vi "GetDeviceModel.vi"(8 "error in (no error)":errorcluster) -> (0 "error out":errorcluster, 1 "found":bool, 3 "device model":T1)   [LabVIEW 2017, in "GlobalConfiguration.lvlib"]
doc: "Returns the entire device model, including device properties, channel properties, and tags."
uses:
  <vilib>/addons/InsightCM/Utilities/GlobalConfiguration/GlobalConfiguration.lvlib
  <vilib>/addons/InsightCM/MessageBus/Base/controls/R2_DeviceModel.ctl
  <vilib>/addons/InsightCM/MessageBus/Base/controls/R2_Device.ctl
  <vilib>/addons/InsightCM/MessageBus/Base/controls/KeyValuePair.ctl
  <vilib>/addons/InsightCM/MessageBus/Base/controls/DeviceState.ctl
  <vilib>/addons/InsightCM/MessageBus/Base/controls/R2_DataGroup.ctl
  <vilib>/addons/InsightCM/MessageBus/Base/controls/OperatingState.ctl
  <vilib>/addons/InsightCM/MessageBus/Base/controls/Trigger.ctl
  <vilib>/addons/InsightCM/MessageBus/Base/controls/Condition.ctl
  <vilib>/addons/InsightCM/MessageBus/Base/controls/BurstModeTrigger.ctl
  <vilib>/addons/InsightCM/MessageBus/Base/controls/DeviceSensorGroup.ctl
  <vilib>/addons/InsightCM/MessageBus/Base/controls/Endpoint.ctl
  <vilib>/addons/InsightCM/MessageBus/Base/controls/WirelessChannel.ctl
  <vilib>/addons/InsightCM/MessageBus/Base/controls/R2_Channel.ctl
  <vilib>/addons/InsightCM/MessageBus/Base/controls/Metric.ctl
  <vilib>/addons/InsightCM/MessageBus/Base/controls/Tag.ctl
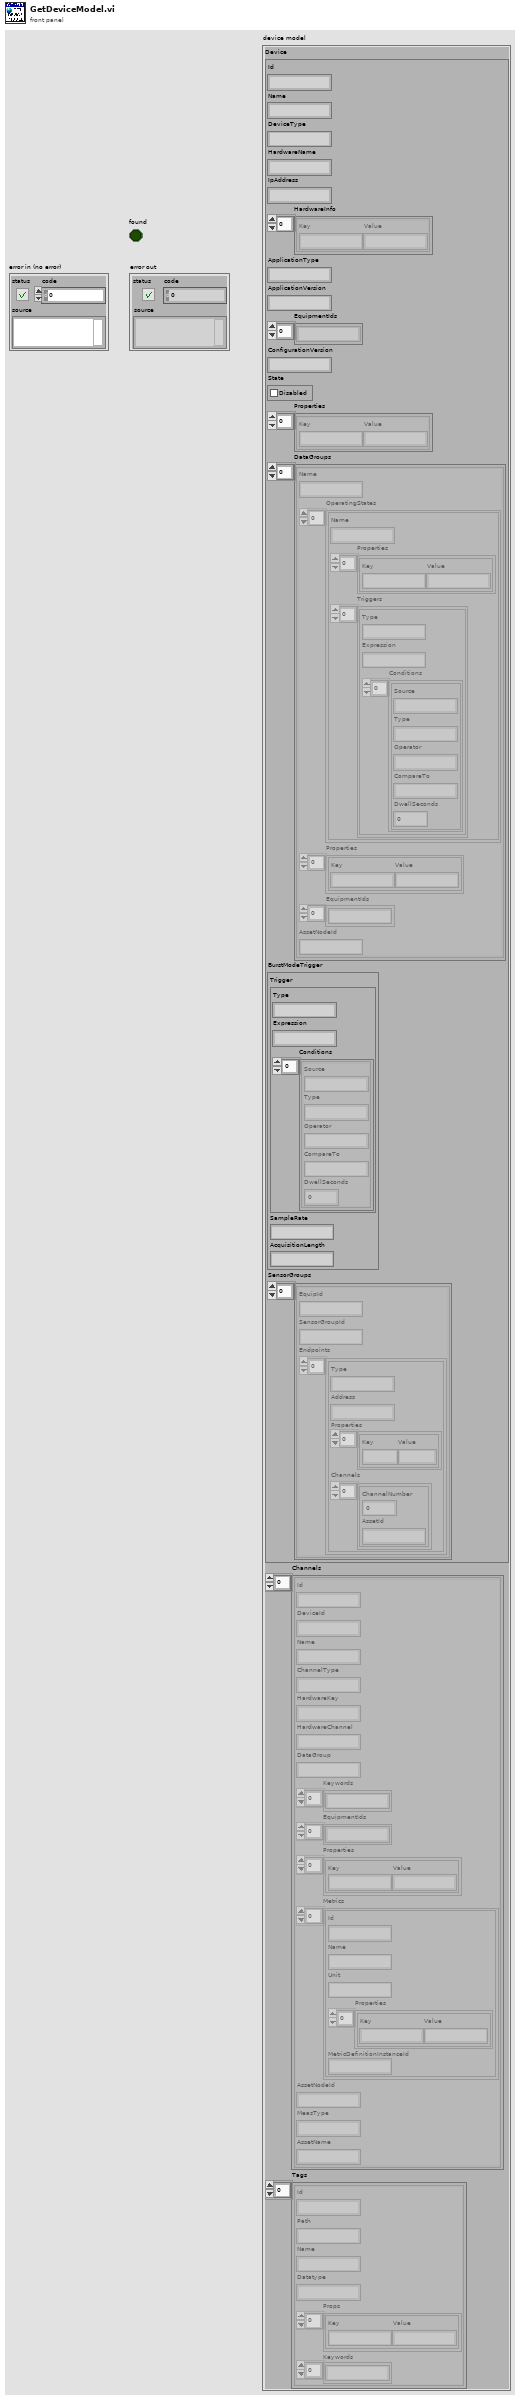
[diagram p1: front panel]
types:
  T1 = typedef "R2_DeviceModel.ctl" = cluster{"Device":T2, "Channels":T13[], "Tags":T15[]}
  T2 = typedef "R2_Device.ctl" = cluster{"Id":string, "Name":string, "DeviceType":string, "HardwareName":string, "IpAddress":string, "HardwareInfo":T3[], "ApplicationType":string, "ApplicationVersion":string, "EquipmentIds":string[], "ConfigurationVersion":string, "State":T4, "Properties":T3[], "DataGroups":T5[], "BurstModeTrigger":T9, "SensorGroups":T10[]}
  T3 = typedef "KeyValuePair.ctl" = cluster{"Key":string, "Value":string}
  T4 = typedef "DeviceState.ctl" = cluster{"Disabled":bool}
  T5 = typedef "R2_DataGroup.ctl" = cluster{"Name":string, "OperatingStates":T6[], "Properties":T3[], "EquipmentIds":string[], "AssetNodeId":string}
  T6 = typedef "OperatingState.ctl" = cluster{"Name":string, "Properties":T3[], "Triggers":T7[]}
  T7 = typedef "Trigger.ctl" = cluster{"Type":string, "Expression":string, "Conditions":T8[]}
  T8 = typedef "Condition.ctl" = cluster{"Source":string, "Type":string, "Operator":string, "CompareTo":string, "DwellSeconds":dbl}
  T9 = typedef "BurstModeTrigger.ctl" = cluster{"Trigger":T7, "SampleRate":string, "AcquisitionLength":string}
  T10 = typedef "DeviceSensorGroup.ctl" = cluster{"EquipId":string, "SensorGroupId":string, "Endpoints":T11[]}
  T11 = typedef "Endpoint.ctl" = cluster{"Type":string, "Address":string, "Properties":T3[], "Channels":T12[]}
  T12 = typedef "WirelessChannel.ctl" = cluster{"ChannelNumber":i32, "AssetId":string}
  T13 = typedef "R2_Channel.ctl" = cluster{"Id":string, "DeviceId":string, "Name":string, "ChannelType":string, "HardwareKey":string, "HardwareChannel":string, "DataGroup":string, "Keywords":string[], "EquipmentIds":string[], "Properties":T3[], "Metrics":T14[], "AssetNodeId":string, "MeasType":string, "AssetName":string}
  T14 = typedef "Metric.ctl" = cluster{"Id":string, "Name":string, "Unit":string, "Properties":T3[], "MetricDefinitionInstanceId":string}
  T15 = typedef "Tag.ctl" = cluster{"Id":string, "Path":string, "Name":string, "Datatype":string, "Props":T3[], "Keywords":string[]}
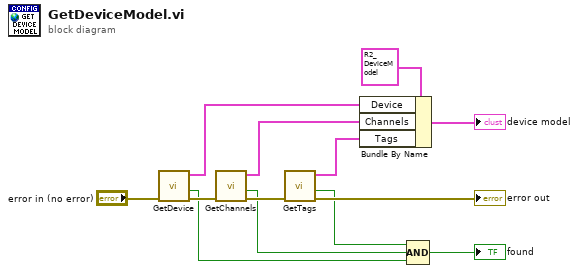
[diagram p0: block diagram]
diagram:
  n1 = call <vilib>:"GetDevice.vi"("error in (no error)"="error in (no error)") -> ("error out"=w10:errorcluster, "found"=w4:bool, "device configuration"=w7:T2)  [unwired: 8 in]
  n2 = call <vilib>:"GetChannels.vi"("error in (no error)"=w10) -> ("error out"=w9:errorcluster, "found"=w3:bool, "channels"=w6:T13[])  [unwired: 8 in]
  n3 = call <vilib>:"GetTags.vi"("error in (no error)"=w9) -> ("error out"=→"error out":errorcluster, "found"=w2:bool, "tags"=w5:T15[])  [unwired: 8 in]
  n4 = Bundle By Name(cluster=T1 {"Device"={"Id"="", "Name"="", "DeviceType"="", "HardwareName"="", "IpAddress"="", "HardwareInfo"=[], "ApplicationType"="", "ApplicationVersion"="", "EquipmentIds"=[], "ConfigurationVersion"="", "State"={"Disabled"=FALSE}, "Properties"=[], "DataGroups"=[], "BurstModeTrigger"={"Trigger"={"Type"="", "Expression"="", "Conditions"=[]}, "SampleRate"="", "AcquisitionLength"=""}, "SensorGroups"=[]}, "Channels"=[], "Tags"=[]} ("DeviceModel"), "Device"=w7, "Channels"=w6, "Tags"=w5) -> (→"device model":T1)
  n5 = Compound Arithmetic op=AND(w2, w3, w4) -> (→"found":bool)
